vi "setCalParameters.vi"(4 "calType":enum16{"INTERNAL_CAL", "FULL_CAL"}(ring), 6 "pdlCal?":u8, 7 "measType":u8, 8 "deciFactor":u32, 9 "numAvgs":u32, 10 "endWL":dbl format="%.2f", 11 "startWL":dbl format="%.2f") -> ()   [LabVIEW 2024]
uses:
  Program Files (x86)/Luna Technologies/OVA 5000 v5.14.2/data/OVA32.dll
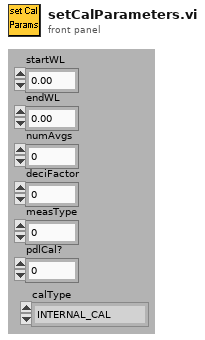
[diagram p1: front panel]
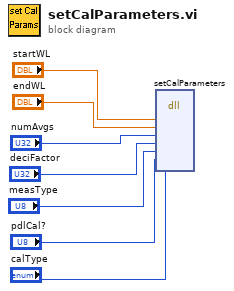
[diagram p0: block diagram]
diagram:
  n1 = dll-call lib="C:/Program Files (x86)/Luna Technologies/OVA 5000 v5.14.2/data/OVA32.dll" fn="setCalParameters"("startWL"="startWL", "endWL"="endWL", "numAvgs"="numAvgs", "deciFactor"="deciFactor", "measType"="measType", "pdlCal"="pdlCal?", "calType"="calType") -> ()  [unwired: 11 in, 2 out]
